vi "Quit GNU Octave.vi"(8 "error in":errorcluster, 11 "GOLPI ref. in":T1={"pipe handle"={"lv_proc.dll file path"=path "", "process instance handle"=[], "debug mode"=FALSE, "debug data"=[]}, "fast read timeout [ms]"=500, "fast read settle time [ms]"=10, "fast read to multiple [ms]"=1, "max elements per input line"=100, "slow read timeout [ms]"=5000, "stdin double format specifier"="%_16e", "max elements per stdout output column"=100, "console mode bitstream"=FALSE, "bitstream first read timeout [ms]"=1000, "bitstream read timeout [ms]"=50, "struct transfer possible"=FALSE, "matlab mode"=FALSE}) -> (0 "error out":errorcluster, 2 "exit code":i32)   [LabVIEW 2020, in "GOLPI library.lvlib"]
doc: "Quits GNU Octave by any means. First sends command 'exit', if not sucessfull closes or kills the GNU Octave process.\n\n---\nGOLPI works only with lv_proc.dll library, which is part of vipm package or should be delivered together with packed library. Placement of this dll is selected in terminal of Start GNU Octave.vi."
uses:
  GOLPI library.lvlib
  GOLPI reference Type Def.ctl
  Pipe Handle.ctl
  LV Process library.lvlib
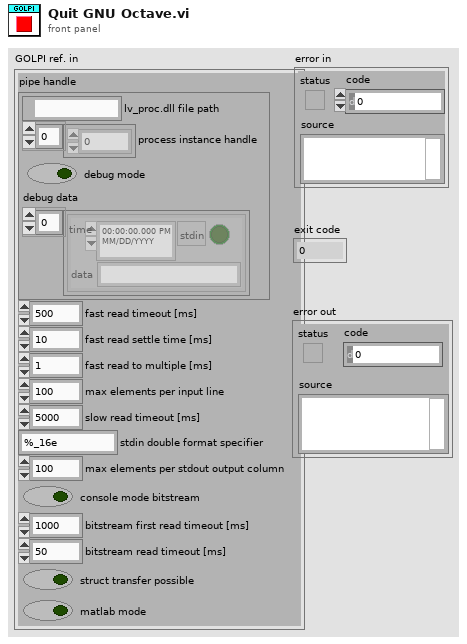
[diagram p1: front panel]
types:
  T1 = typedef "GOLPI library.lvlib/GOLPI reference Type Def.ctl" = cluster{"pipe handle":T2, "fast read timeout [ms]":u32, "fast read settle time [ms]":u32, "fast read to multiple [ms]":u32, "max elements per input line":u32, "slow read timeout [ms]":u32, "stdin double format specifier":string, "max elements per stdout output column":u32, "console mode bitstream":bool, "bitstream first read timeout [ms]":u32, "bitstream read timeout [ms]":u32, "struct transfer possible":bool, "matlab mode":bool}
  T2 = typedef "LV Process library.lvlib/Pipe Handle.ctl" = cluster{"lv_proc.dll file path":path, "process instance handle":u32[], "debug mode":bool, "debug data":cluster{"time":timestamp, "stdin":bool, "data":string}[]}
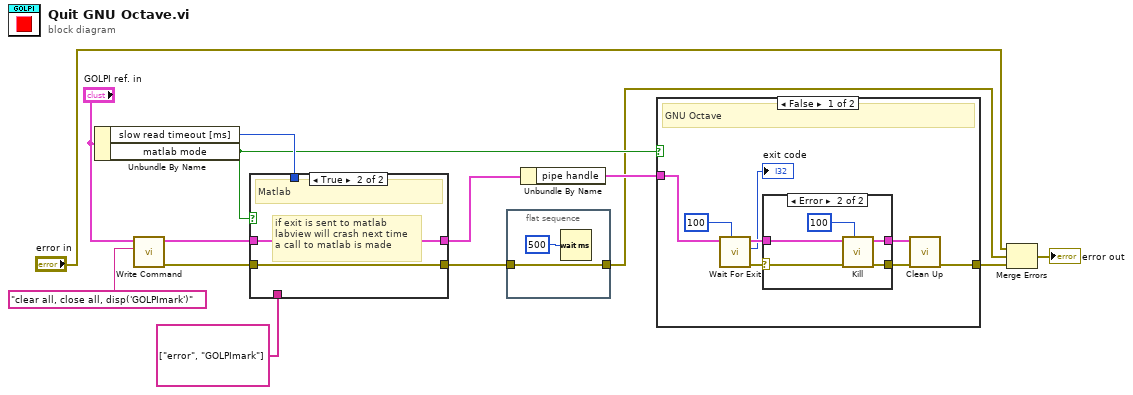
[diagram p0: block diagram]
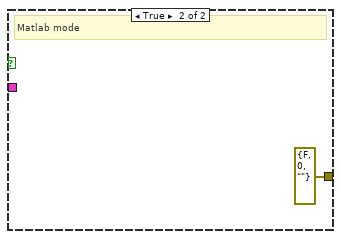
[diagram p3: hidden frame]
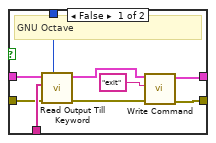
[diagram p4: hidden frame]
diagram:
  n1 = Unbundle By Name("GOLPI ref. in") -> ("slow read timeout [ms]"=w8:u32, "matlab mode"=w7:bool)
  n2 = call "Write Command.vi"("command"="clear all, close all, disp('GOLPImark')" ("write buffer"), "GOLPI ref. in"="GOLPI ref. in") -> ("error out"=w12:errorcluster, "GOLPI ref. out"=w11:T1)  [unwired: 8 in]
  n3 = case shown="True" w7 {
    tunnel: string[] ["error", "GOLPImark"] ("keywords") -> [w23 _]
    tunnel: w12 -> [w22 w25]
    tunnel: w11 -> [w21 w24]
    tunnel: [w15 w24] -> w2
    tunnel: [w18 w25] -> w1
    tunnel: w8 -> [w20 _]
    frame False {
      # "GNU Octave"
      n4 = call "Read Output Till Keyword.vi"("timeout [ms]"=w20, "error in"=w22, "keywords"=w23, "GOLPI ref. in"=w21) -> ("error out"=w17:errorcluster, "GOLPI ref. out"=w16:T1)  [unwired: 4 in, 2 out]
      n5 = call "Write Command.vi"("error in"=w17, "command"="exit", "GOLPI ref. in"=w16) -> ("error out"=w18:errorcluster, "GOLPI ref. out"=w15:T1)  [unwired: 7 in]
    }
    frame True {
      # "if exit is sent to matlab\nlabview will crash next time\na call to matlab is made"
      # "Matlab"
    }
  }
  n6 = flat-sequence {
    tunnel: [w26] -> w4
    tunnel: w1 -> [w26]
    frame #0 {
      n7 = Wait (ms)(milliseconds to wait=u32 500) -> ()  [unwired: 1 out]
    }
  }
  n8 = Unbundle By Name(w2) -> ("pipe handle"=w10:T2)
  n9 = case shown="False" w7 {
    tunnel: [w35 errorcluster {"status"=FALSE, "code"=0, "source"=""} ("error out")] -> w6
    tunnel: w10 -> [w28 _]
    frame False {
      # "GNU Octave"
      n10 = call "Wait For Exit.vi"("timeout [ms] (1)"=100 ("timeout [ms]"), "pipe in"=w28) -> ("error out"=w33:errorcluster, "exit code"=→"exit code":i32, "pipe out"=w32:T2)  [unwired: 7 in]
      n11 = case shown="Error" w33 {
        selector: w33 -> [w36 w41]
        tunnel: w32 -> [w37 w40]
        tunnel: [w36 w42] -> w34
        tunnel: [w37 w39] -> w30
        frame No Error {
        }
        frame Error {
          n12 = call "Kill.vi"("timeout [ms]"=100, "error in"=w41, "pipe in"=w40) -> ("error out"=w42:errorcluster, "pipe out"=w39:T2)  [unwired: 7 in]
        }
      }
      n13 = call "Clean Up.vi"("error in"=w34, "pipe in"=w30) -> ("error out"=w35:errorcluster)  [unwired: 9 in]
    }
    frame True {
      # "Matlab mode"
    }
  }
  n14 = Merge Errors("error in", w4, w6) -> (→"error out":errorcluster)
